vi "Number to String Array.vi"(9 "number":dbl[](array[numeric]), 10 "Board Info":string) -> (2 "Output Array":string[](array[string]))   [LabVIEW 2016, in "Data Saving.lvlib" / "Excel Saver.lvclass"]
uses:
  Excel Saver.lvclass
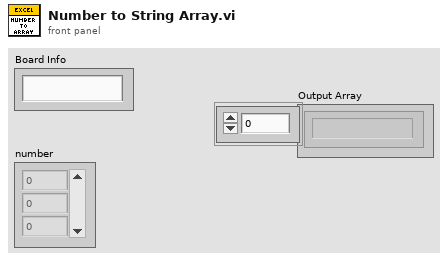
[diagram p1: front panel]
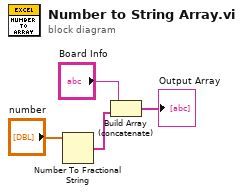
[diagram p0: block diagram]
diagram:
  n1 = Number To Fractional String(number="number") -> (F-format string=w4:string[])  [unwired: 3 in]
  n2 = Build Array (concatenate)("Board Info", w4) -> (→"Output Array":string[])
